vi "test_Placeholder (Zero) Argument (One).vi"(8 "error in (no error)":errorcluster, 11 "TestCase in":refnum<class "Test JSON Layout.lvclass">) -> (0 "error out":errorcluster, 3 "TestCase out":refnum<class "Test JSON Layout.lvclass">)   [LabVIEW 2019, in "Test JSON Layout.lvclass"]
uses:
  Test JSON Layout.lvclass
  C:/Program Files/National Instruments/LabVIEW 2024/vi.lib/Astemes/LUnit/Test Case.lvclass
  <vilib>/Astemes/LUnit/Test Case.lvclass/Test Case.ctl
  9fa21a26-ce0f-4c3d-8adb-95555ae4ffb5.vi
  <vilib>/Astemes/LUnit/Core/LUnit Test Case/Private/Append Pass Result.vi
  <vilib>/Astemes/LUnit/Core/LUnit Test Case/Private/Append Fail Result.vi
  9fa21a26-ce0f-4c3d-8adb-95555ae4ffb5.vi/9c5d11cd-9439-4240-a1ee-d9baace9c924.vi
  <vilib>/Astemes/LUnit/Core/LUnit Test Case/Private/Run In UI.vi
  <vilib>/Utility/error.llb/Clear Errors.vi
  Layouts/JSONLayout/JSONLayout.lvclass
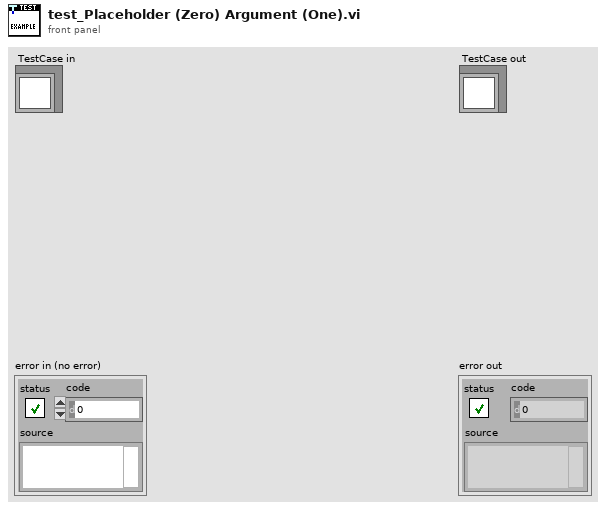
[diagram p1: front panel]
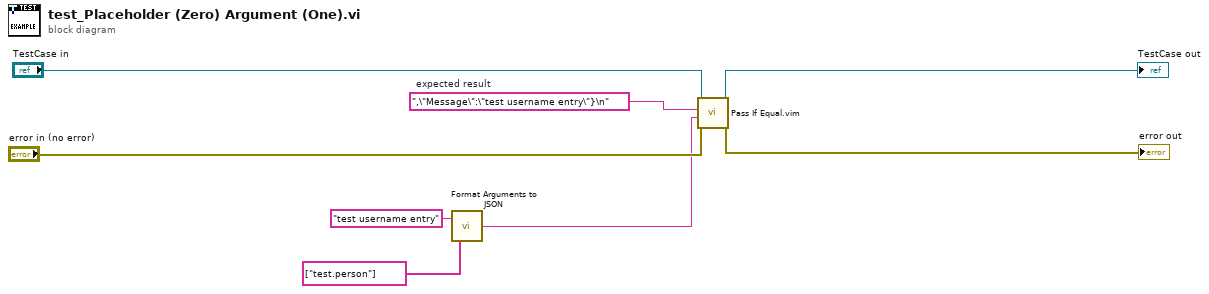
[diagram p0: block diagram]
diagram:
  w4 = ",\"Message\":\"test username entry\"}\n"  # expected result
  n1 = call "Format Arguments to JSON.vi"("Arguments"=string[] ["test.person"], "Message"="test username entry") -> ("Output Message"=w1:string)
  n2 = call "Pass If Equal.vim"("error in (no error)"="error in (no error)", "Actual"=w1, "Expected"=w4, "LUnit Test Case In"="TestCase in") -> ("error out"=→"error out":errorcluster, "LUnit Test Case Out"=→"TestCase out":refnum<class "Test JSON Layout.lvclass">)  [unwired: 6 in]
